vi "FTW-Endpoint-Core-Ask.vi"(0 "FTW Socket":refnum<class "FTW-Endpoint.lvclass">, 5 "Request":string, 7 "Read Timeout":i32=100 format="%dmsec", 9 "Write Timeout":i32 format="%dmsec", 11 "error in":errorcluster) -> (4 "FTW Socket out":refnum<class "FTW-Endpoint.lvclass">, 6 "Response":string, 8 "Read Timed out?":bool, 10 "Write Timed out?":bool, 15 "error out":errorcluster)   [LabVIEW 2012, in "FTW-Actor.lvlib" / "FTW-Endpoint.lvclass"]
uses:
  FTW-Endpoint.lvclass
  FTW-Endpoint.lvclass/FTW-Endpoint.ctl
panel:
  out "x = y?":bool
  # "Inputs"
  # "Outputs"
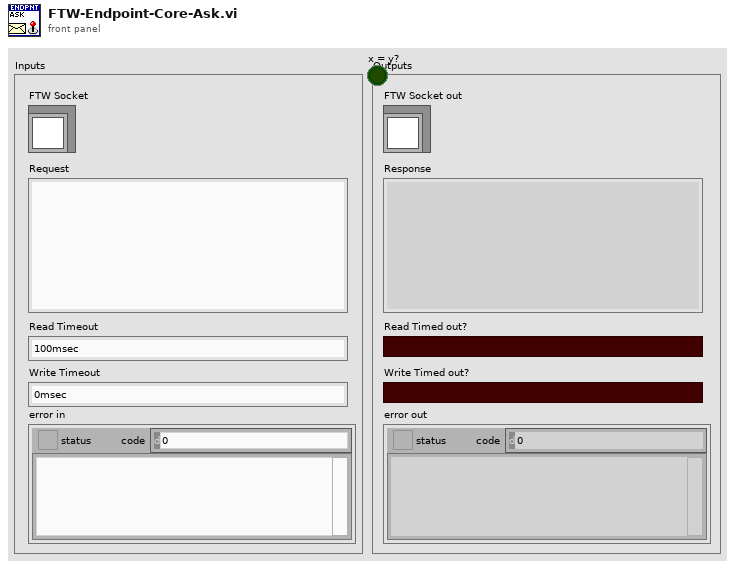
[diagram p1: front panel]
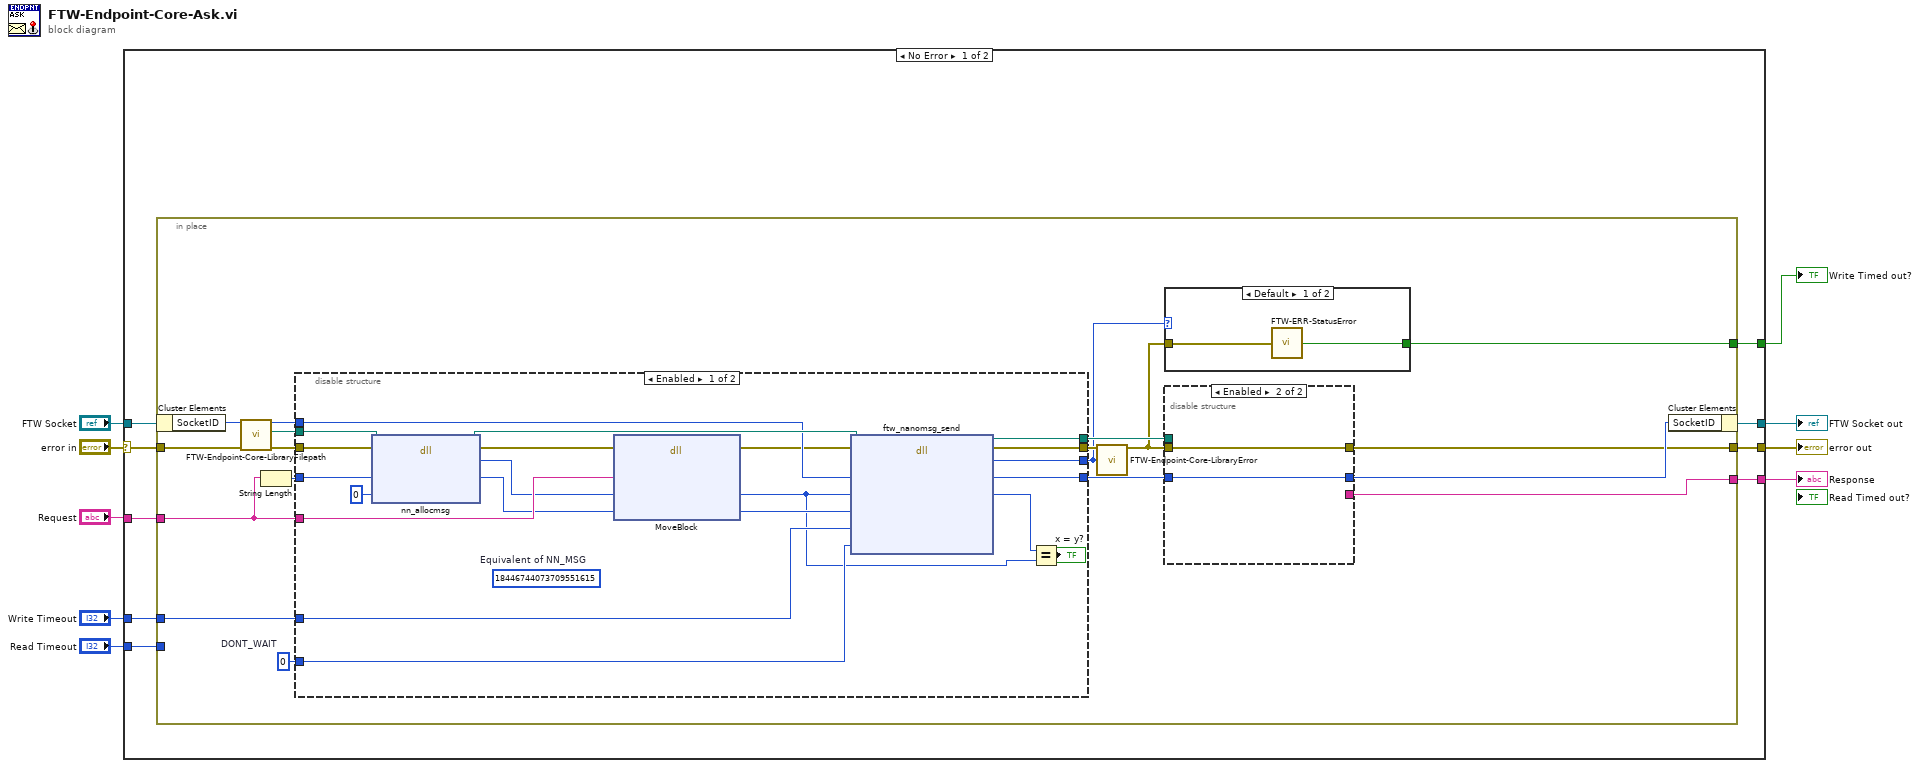
[diagram p0: block diagram]
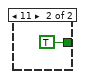
[diagram p2: hidden frame]
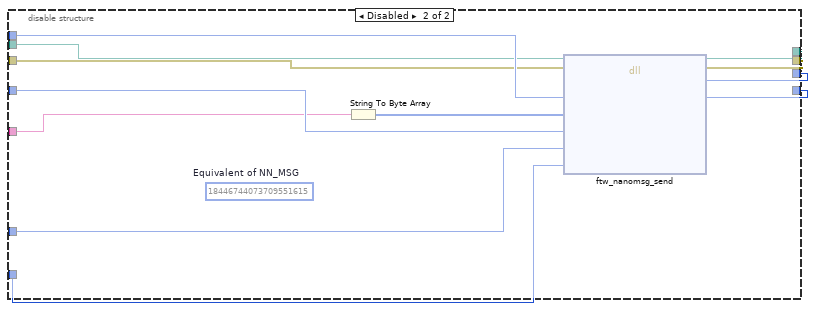
[diagram p3: hidden frame]
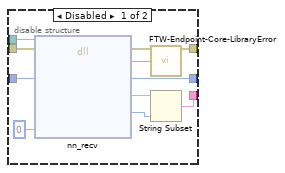
[diagram p4: hidden frame]
diagram:
  n1 = case shown="No Error" "error in" {
    selector: "error in" -> [w14 w85]
    tunnel: "FTW Socket" -> [w18 w86]
    tunnel: "Request" -> [w17 _]
    tunnel: [w16 w85] -> w4
    tunnel: [w15 w86] -> w5
    tunnel: "Read Timeout" -> [w13 _]
    tunnel: [w12 _] -> w3
    tunnel: "Write Timeout" -> [w11 _]
    tunnel: [w10 _] -> w1
    frame No Error {
      n2 = in-place {
        in-place-border: w17 -> [w34]
        in-place-border: w14 -> [w31]
        in-place-border: [w28] -> w16
        in-place-border: w13 -> [_]
        in-place-border: [w32] -> w12
        in-place-border: w11 -> [w27]
        in-place-border: [w19] -> w10
        w23 = 0  # DONT_WAIT
        n3 = in-place-cluster #1(w18) -> ("SocketID"=w35:i64)
        n4 = call "FTW-Endpoint-Core-LibraryFilepath.vi"("error in"=w31) -> ("error out"=w30:errorcluster, "Library Filepath"=w29:path)  [unwired: 8 in, 1 out]
        n5 = String Length(string=w34) -> (length=w22:i32)
        n6 = disable-structure shown="Enabled" {
          disable-tunnel: w34 -> [w59 w61]
          disable-tunnel: w22 -> [w58 w62]
          disable-tunnel: w30 -> [w53 w63]
          disable-tunnel: w29 -> [w52 w64]
          disable-tunnel: w35 -> [w49 w71]
          disable-tunnel: w27 -> [w48 w70]
          disable-tunnel: w23 -> [w47 w69]
          disable-tunnel: [w45 w68] -> w24
          disable-tunnel: [w44 w67] -> w26
          disable-tunnel: [w43 w66] -> w21
          disable-tunnel: [w42 w65] -> w25
          frame Enabled {
            (unwired) u64 18446744073709551615  # Equivalent of NN_MSG
            n7 = dll-call lib="?" fn="nn_allocmsg"(path in=w52, error in=w53, "Message Size"=w58, "Message Type"=0 ("type")) -> (path out=w51:path, error out=w55:errorcluster, "Return Value"=w56:i64, "Message Size"=w54:i32)  [unwired: 2 in]
            n8 = dll-call lib="LabVIEW" fn="MoveBlock"(error in=w55, "Source String"=w59, "Pointer to Destination"=w56, "String Length"=w54) -> (error out=w46:errorcluster, "Pointer to Destination"=w40:i64, "String Length"=w50:i32)  [unwired: 4 in, 1 out]
            n9 = dll-call lib="?" fn="ftw_nanomsg_send"(path in=w51, error in=w46, "SocketID"=w49, "Message"=w40, "Length"=w50, "Timeout"=w48, "Flags"=w47) -> (path out=w45:path, error out=w44:errorcluster, "Return Value"=w43:i64, "SocketID"=w42:i64, "Message"=w41:i64)  [unwired: 4 in]
            n10 = Equal?(x=w41, y=w40) -> (x = y?=→"x = y?":bool)
          }
          frame Disabled {
            (unwired) u64 18446744073709551615  # Equivalent of NN_MSG
            n11 = String To Byte Array(string=w61) -> (unsigned byte array=w60:u8[])
            n12 = dll-call lib="?" fn="ftw_nanomsg_send"(path in=w64, error in=w63, "SocketID"=w71, "Message"=w60, "Length"=w62, "Timeout"=w70, "Flags"=w69) -> (path out=w68:path, error out=w67:errorcluster, "Return Value"=w66:i64, "SocketID"=w65:i64)  [unwired: 5 in]
          }
        }
        n13 = call "FTW-Endpoint-Core-LibraryError.vi"("error in"=w26, "Return Value"=w21) -> ("error out"=w20:errorcluster)  [unwired: 13 in]
        n14 = case shown="Default" w21 {
          tunnel: w20 -> [w37 _]
          tunnel: [w36 TRUE ("Status OK?")] -> w19
          frame Default {
            n15 = call "FTW-ERR-StatusError.vi"("error to check"=w37) -> ("Error?"=w36:bool)
          }
          frame 11 {
          }
        }
        n16 = disable-structure shown="Enabled" {
          disable-tunnel: w25 -> [w80 w83]
          disable-tunnel: [w79 w83] -> w33
          disable-tunnel: [w77 _] -> w32
          disable-tunnel: w20 -> [w74 w84]
          disable-tunnel: w24 -> [w73 _]
          disable-tunnel: [w72 w84] -> w28
          frame Disabled {
            n17 = dll-call lib="?" fn="nn_recv"(path in=w73, error in=w74, "SocketID"=w80, "Flags"=0) -> (error out=w82:errorcluster, "Return Value"=w81:i64, "SocketID"=w79:i64, "Message"=w78:string, "Message Length"=w76:u32)  [unwired: 4 in, 1 out]
            n18 = call "FTW-Endpoint-Core-LibraryError.vi"("error in"=w82, "Return Value"=w81) -> ("error out"=w72:errorcluster)  [unwired: 13 in]
            n19 = String Subset(string=w78, length (rest)=w76) -> (substring=w77:string)  [unwired: 1 in]
          }
          frame Enabled {
          }
        }
        n20 = in-place-cluster #1("SocketID"=w33) -> (w15:refnum<class "FTW-Endpoint.lvclass">)
      }
    }
    frame Error {
    }
  }
  "error out" <- w4
  "FTW Socket out" <- w5
  "Response" <- w3
  "Write Timed out?" <- w1
